vi "UI.vi"() -> ()   [LabVIEW 2016, in "中水三立SQL数据传输.lvlib"]
panel:
  out "数据大小":i32
  out "数据上传中":bool
  out "当前时间":timestamp
  out "error out":errorcluster
  out "数据查表起始时间":T1
  in  "数据补传":bool caption="确定"
  out "读取报文显示":string
  out "发送报文显示":string
  out "通信状态":bool
  in  "配置信息":T2
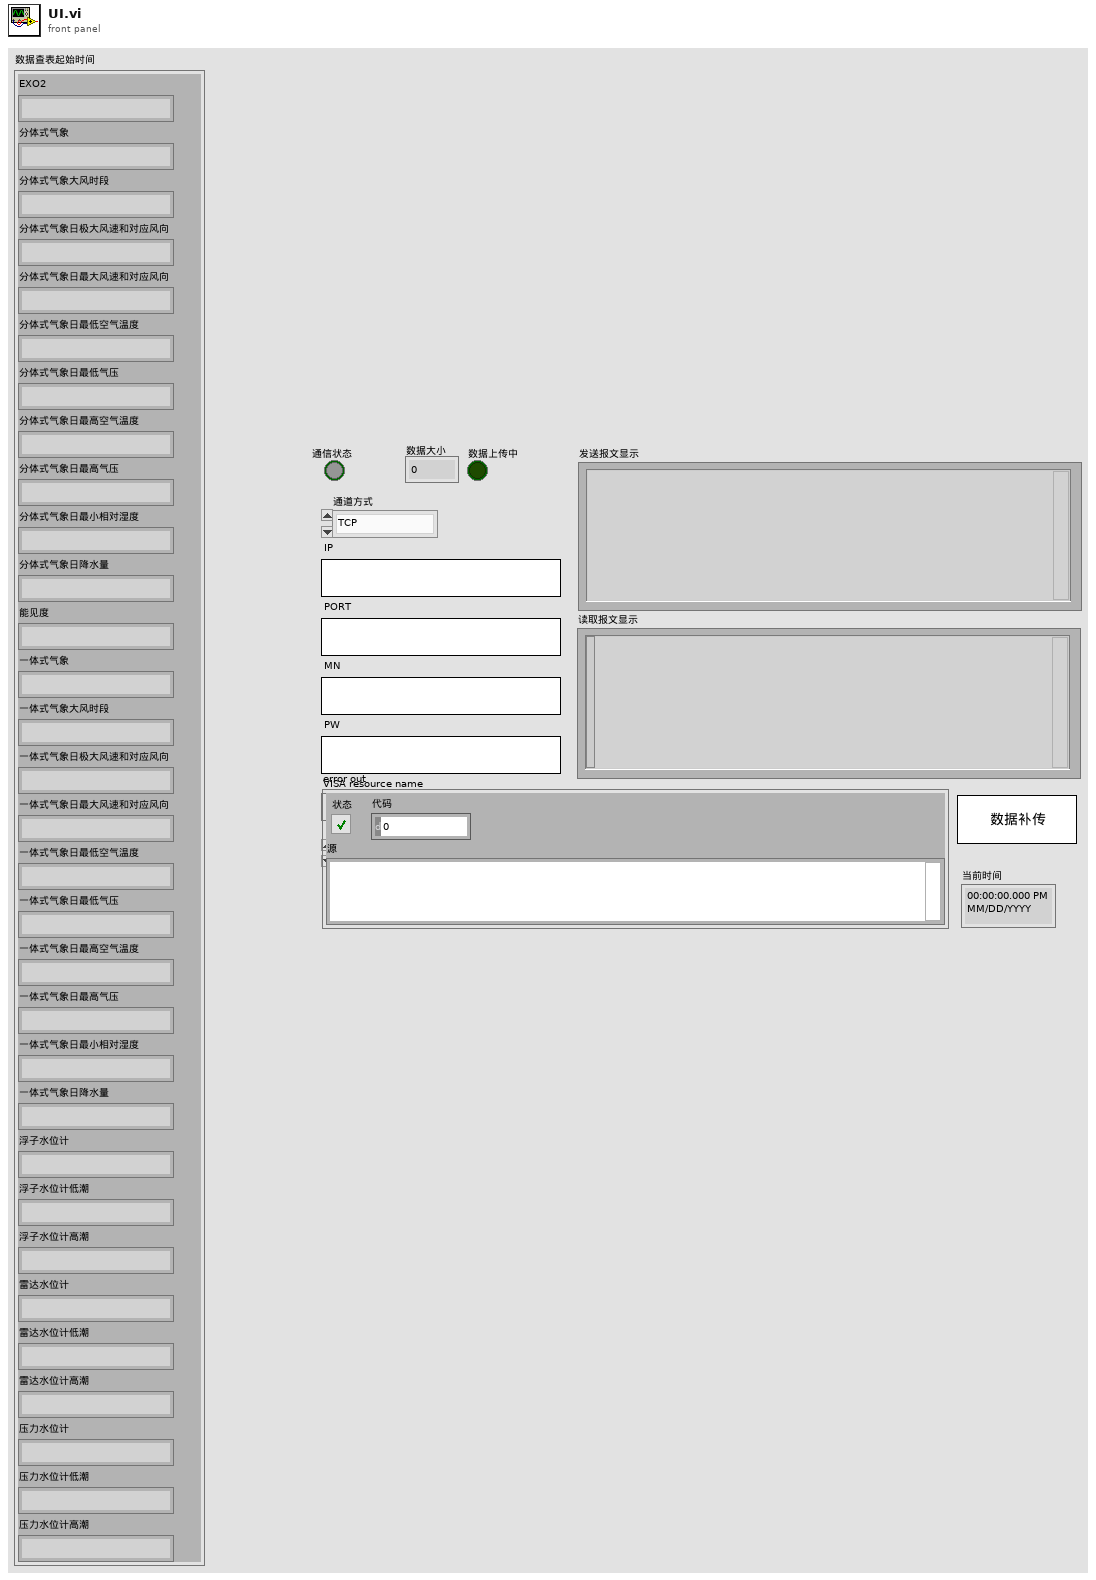
[diagram p1: front panel]
types:
  T1 = cluster{"EXO2":string, "分体式气象":string, "分体式气象大风时段":string, "分体式气象日极大风速和对应风向":string, "分体式气象日最大风速和对应风向":string, "分体式气象日最低空气温度":string, "分体式气象日最低气压":string, "分体式气象日最高空气温度":string, "分体式气象日最高气压":string, "分体式气象日最小相对湿度":string, "分体式气象日降水量":string, "能见度":string, "一体式气象":string, "一体式气象大风时段":string, "一体式气象日极大风速和对应风向":string, "一体式气象日最大风速和对应风向":string, "一体式气象日最低空气温度":string, "一体式气象日最低气压":string, "一体式气象日最高空气温度":string, "一体式气象日最高气压":string, "一体式气象日最小相对湿度":string, "一体式气象日降水量":string, "浮子水位计":string, "浮子水位计低潮":string, "浮子水位计高潮":string, "雷达水位计":string, "雷达水位计低潮":string, "雷达水位计高潮":string, "压力水位计":string, "压力水位计低潮":string, "压力水位计高潮":string}
  T2 = cluster{"通道方式":enum16{"TCP", "serial"}, "IP":string, "PORT":string, "MN":string, "PW":string, "VISA resource name":refnum<visa-resource-name>, "baud rate":u32}
  T3 = typedef "LVDateTimeRec.ctl" = cluster{"秒数的小数部分":dbl, "秒":i32, "分":i32, "时":i32, "日":i32, "月":i32, "年":i32, "天数（周）":i32, "天数（年）":i32, "DST":i32}
  T4 = cluster{"[0]":string, "[1]":string, "[2]":string, "[3]":string, "[4]":string, "[5]":string, "[6]":string, "[7]":string, "[8]":string, "[9]":string, "[10]":string, "[11]":string, "[12]":string, "[13]":string, "[14]":string, "[15]":string, "[16]":string, "[17]":string, "[18]":string, "[19]":string, "[20]":string, "[21]":string, "[22]":string, "[23]":string, "[24]":string, "[25]":string, "[26]":string, "[27]":string, "[28]":string, "[29]":string, "[30]":string}
  T5 = cluster{"枚举":enum16{"TCP", "serial"}, "IP":string, "PORT":string, "MN":string, "PW":string, "VISA resource name":refnum<visa-resource-name>, "baud rate":u32}
  T6 = cluster{"枚举":enum16{"打开连接", "发送数据", "读取数据", "数据处理", "关闭连接"}, "data":string}
  T7 = typedef "中水三立SQL数据传输.lvlib/data_in.ctl" = cluster{"PW":string, "MN":string, "table输入":T8, "数据发送次数":i32, "枚举":enum16{"返回请求应答", "上传数据", "返回执行结果"}, "type":T9, "因子编码&数据类型":cluster{"因子编码":string, "数据类型":string}[]}
  T8 = typedef "中水三立SQL数据传输.lvlib/table.ctl" = string
  T9 = typedef "中水三立SQL数据传输.lvlib/Type.ctl" = string
  T10 = cluster{"table":string, "columns":string[], "condition":string, "data_in":T7}
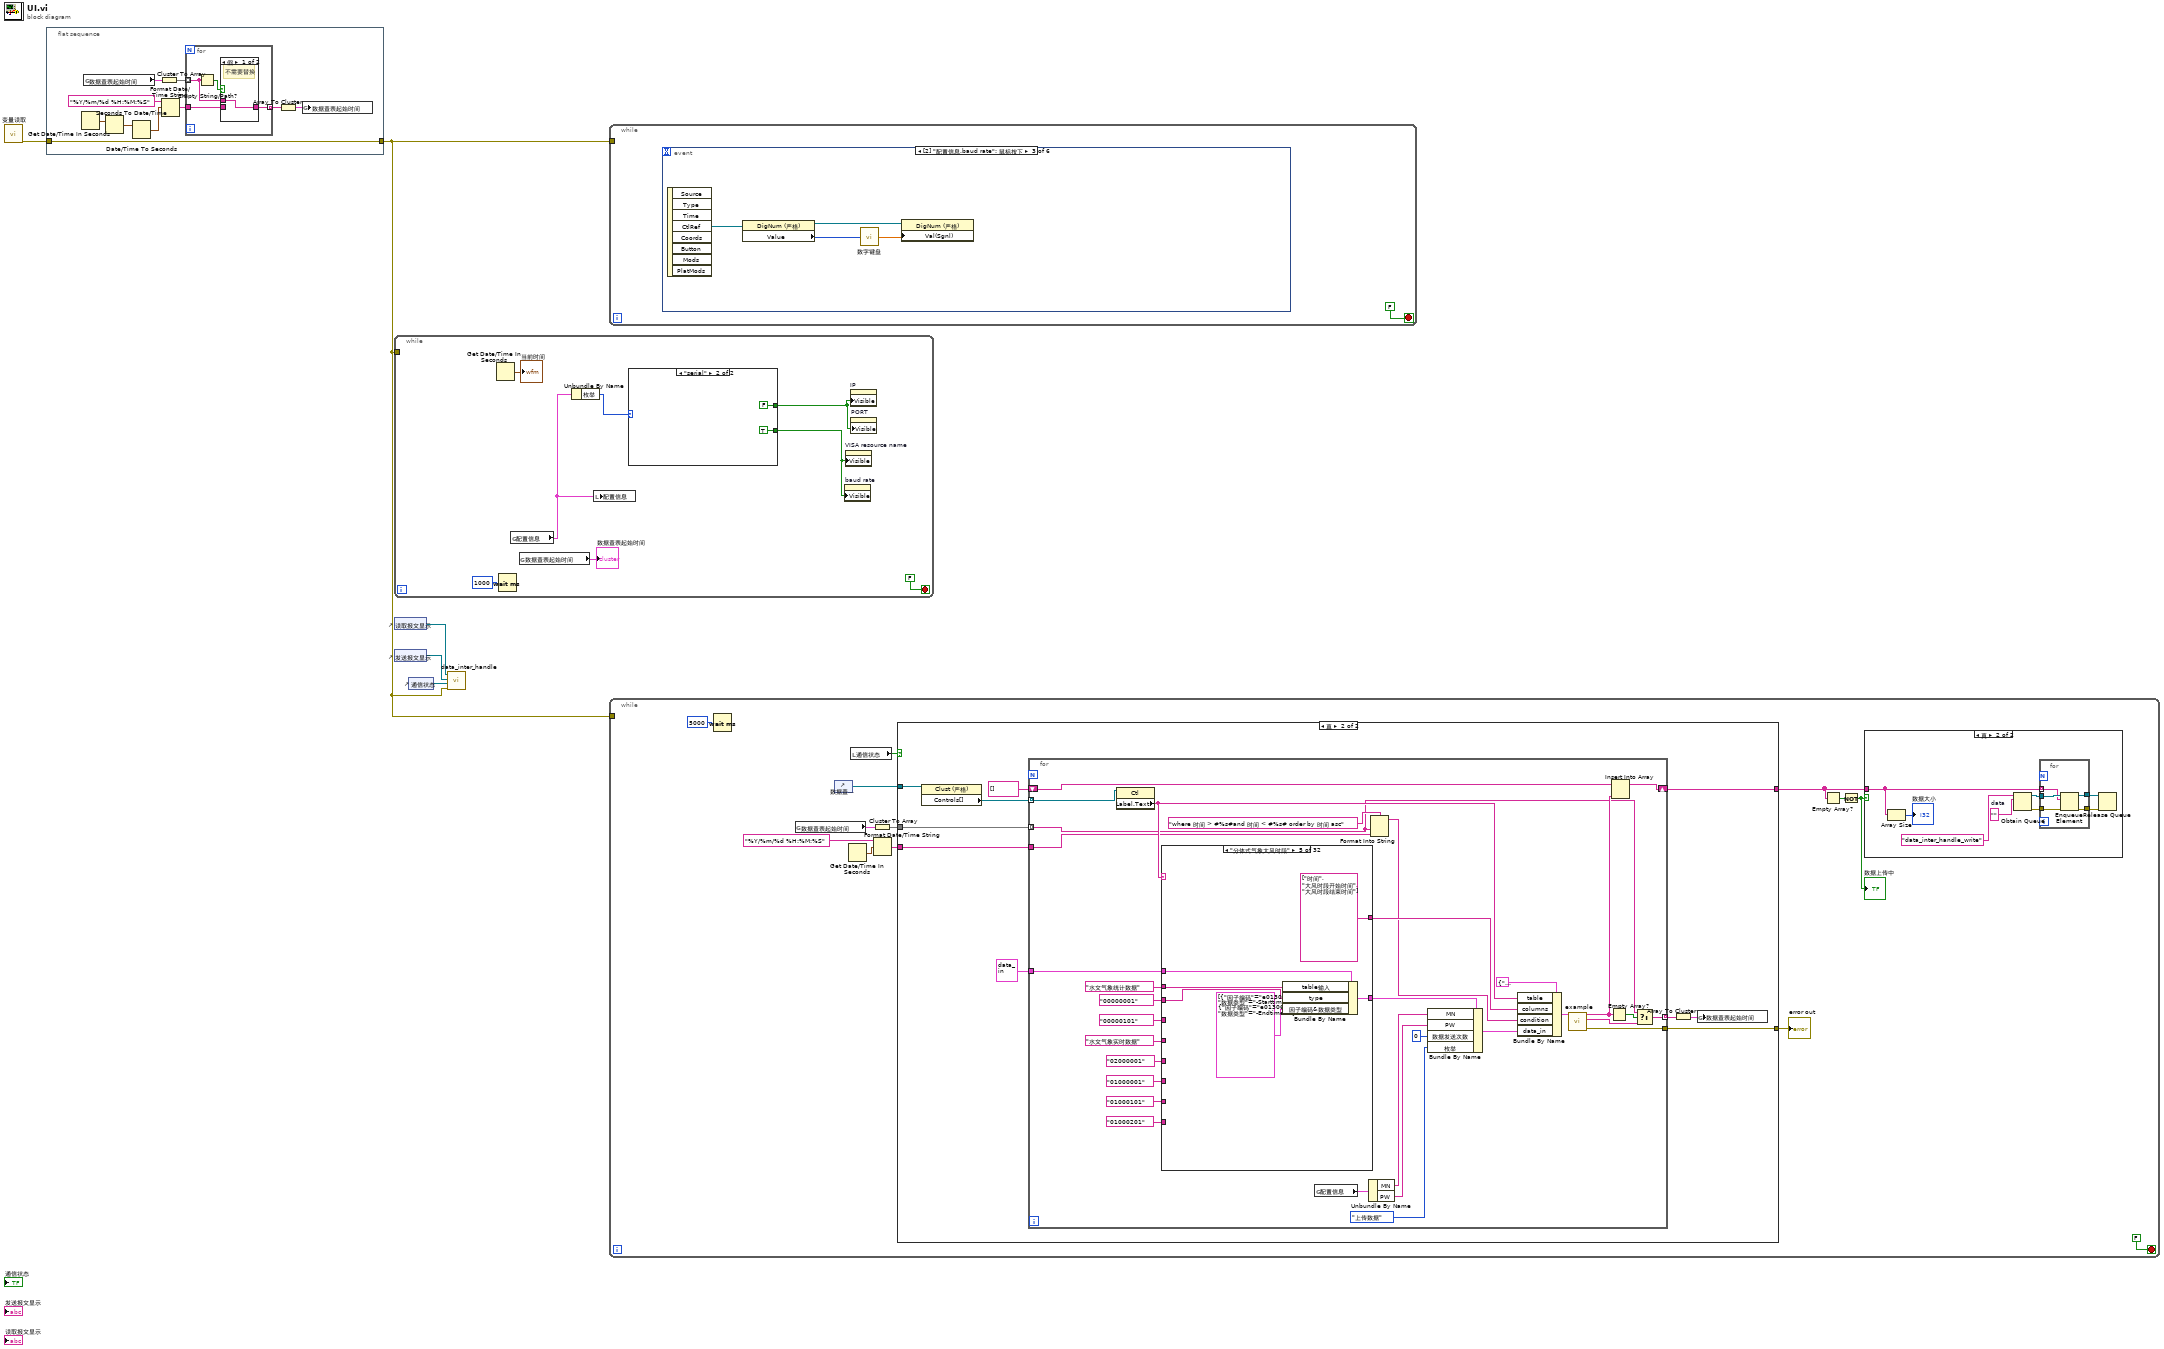
[diagram p0: block diagram]
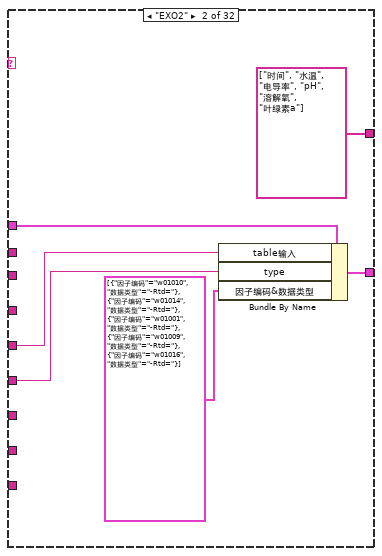
[diagram p5: hidden frame]
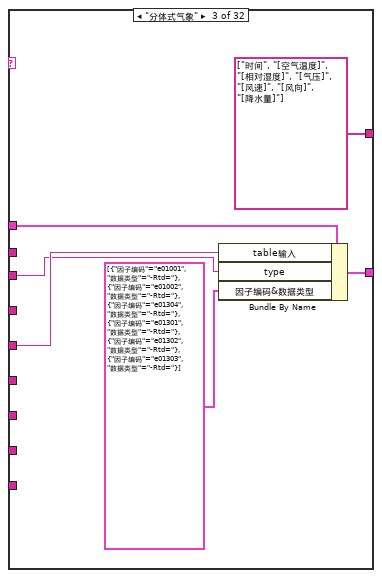
[diagram p6: hidden frame]
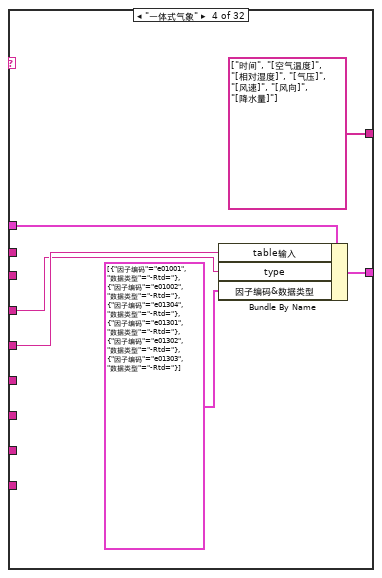
[diagram p7: hidden frame]
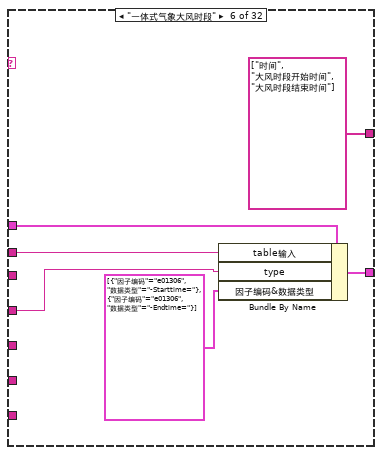
[diagram p8: hidden frame]
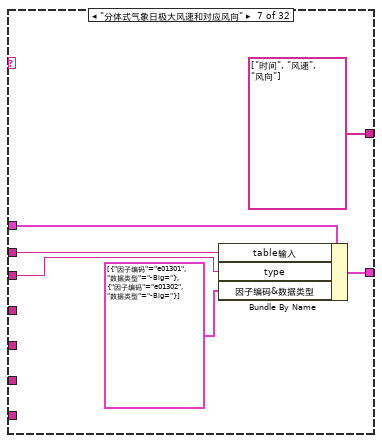
[diagram p9: hidden frame]
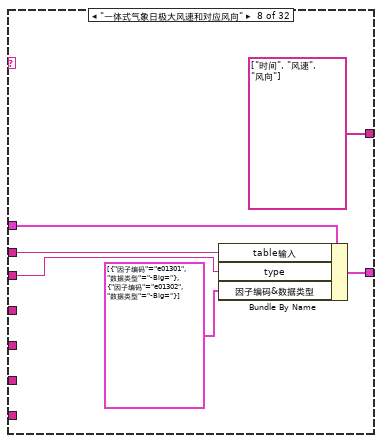
[diagram p10: hidden frame]
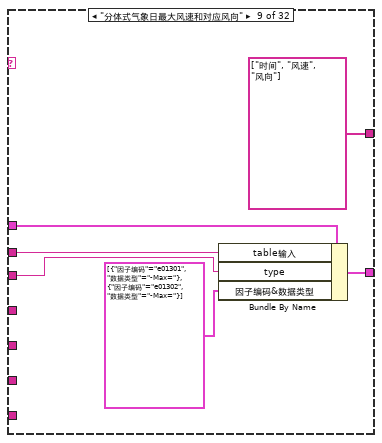
[diagram p11: hidden frame]
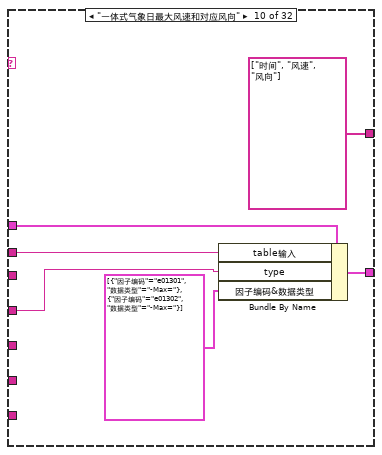
[diagram p12: hidden frame]
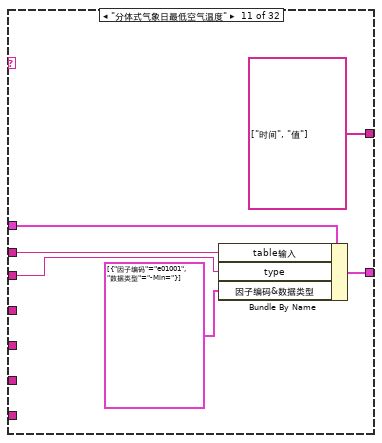
[diagram p13: hidden frame]
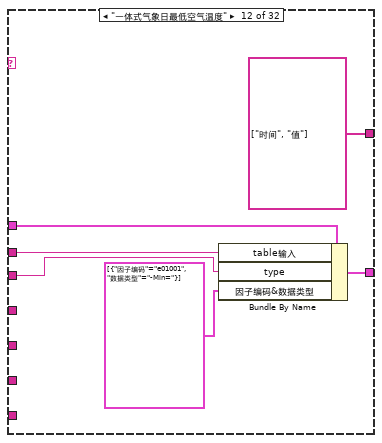
[diagram p14: hidden frame]
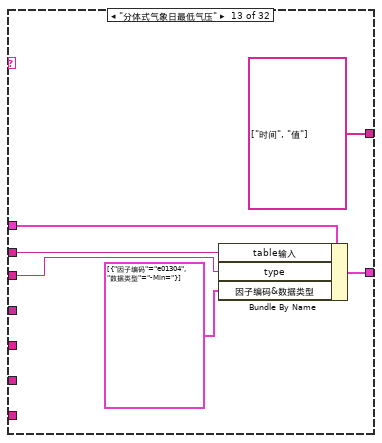
[diagram p15: hidden frame]
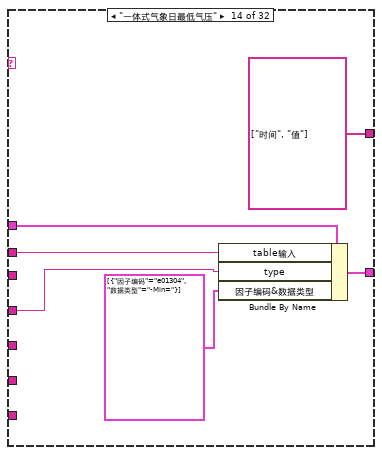
[diagram p16: hidden frame]
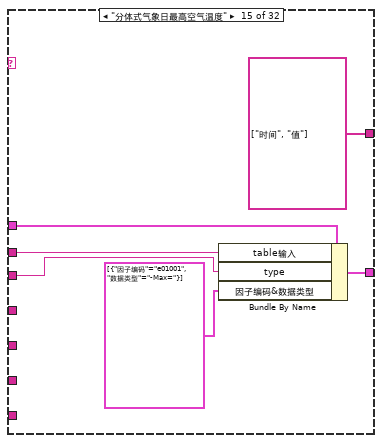
[diagram p17: hidden frame]
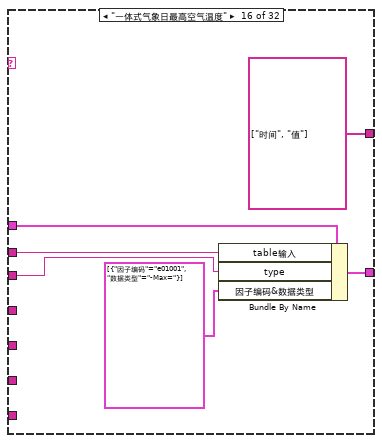
[diagram p18: hidden frame]
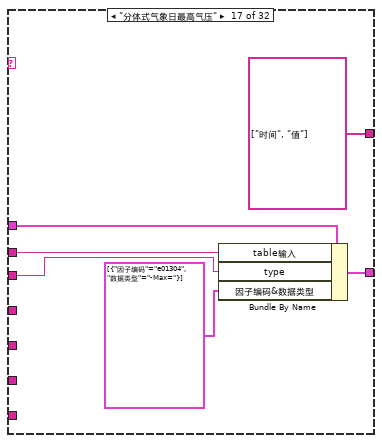
[diagram p19: hidden frame]
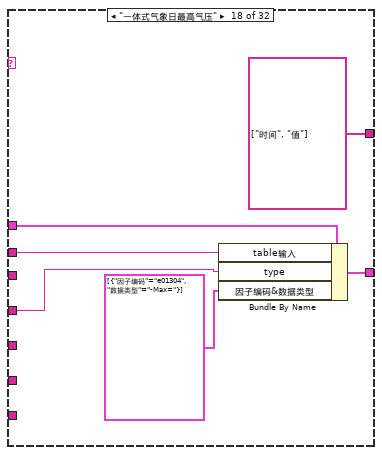
[diagram p20: hidden frame]
diagram:
  n1 = call "变量读取.vi"() -> ("错误输出"=w5:errorcluster)  [unwired: 11 in]
  n2 = flat-sequence {
    tunnel: w5 -> [w8]
    tunnel: [w8] -> w4
    frame #0 {
      n3 = Get Date/Time In Seconds() -> (seconds since 1Jan1904=w7:timestamp)
      n4 = global read "断电保存全局.vi" "数据查表起始时间"() -> (w13:cluster{"dbo.LS_Data":string})
      n5 = Seconds To Date/Time(time stamp (now)=w7) -> (date time rec=w6:T3)  [unwired: 1 in]
      n6 = Date/Time To Seconds(2:w6) -> (0:w11:timestamp)  [unwired: 1 in]
      n7 = Cluster To Array(cluster=w13) -> (array=w14:string[])
      n8 = Format Date/Time String(time format string (%c)="%Y/%m/%d %H:%M:%S" ("时间格式字符串(%c)"), seconds (now)=w11) -> (date/time string=w10:string)  [unwired: 1 in]
      n9 = for {
        tunnel: w14 -> [w16] mode=indexing
        tunnel: w10 -> [w18]
        tunnel: [w17] -> w15 mode=indexing
        n10 = Empty String/Path?(string/path=w16) -> (empty?=w19:bool)
        n11 = case shown="假" w19 {
          tunnel: w18 -> [_ w21]
          tunnel: [w20 w21] -> w17
          tunnel: w16 -> [w20 _]
          frame False {
            # "不需要替换"
          }
          frame True {
            # "空字符串，替换"
          }
        }
      }
      n12 = Array To Cluster(array=w15) -> (cluster=w9:T4)
      n13 = global write "断电保存全局.vi" "数据查表起始时间"(w9) -> ()
    }
  }
  n14 = while {
    tunnel: w4 -> [_]
    stop <- FALSE stop-if-true
    n15 = Get Date/Time In Seconds() -> (seconds since 1Jan1904=→"当前时间":timestamp)
    n16 = Wait (ms)(milliseconds to wait=u32 1000 ("等待时间（毫秒）")) -> ()  [unwired: 1 out]
    n17 = global read "断电保存全局.vi" "配置信息"() -> (w25:T5)
    n18 = global read "断电保存全局.vi" "数据查表起始时间"() -> (→"数据查表起始时间":cluster{"dbo.LS_Data":string})
    n19 = Unbundle By Name(w25) -> ("枚举"=w24:enum16{"TCP", "serial"})
    n20 = local write "配置信息"(w25) -> ()
    n21 = case shown="\"serial\"" w24 {
      tunnel: [TRUE FALSE] -> w23
      tunnel: [FALSE TRUE] -> w22
      frame "TCP", Default {
      }
      frame "serial" {
      }
    }
    n22 = property on="baud rate" class="DigNum (严格)"("Visible"=w22) -> ()  [unwired: 2 in, 2 out]
    n23 = property on="VISA resource name" class="VISAName"("Visible"=w22) -> ()  [unwired: 2 in, 2 out]
    n24 = property on="IP" class="Str"("Visible"=w23) -> ()  [unwired: 2 in, 2 out]
    n25 = property on="PORT" class="Str"("Visible"=w23) -> ()  [unwired: 2 in, 2 out]
  }
  n26 = control-ref of="读取报文显示"() -> (w2:refnum<vi>)
  n27 = control-ref of="发送报文显示"() -> (w3:refnum<vi>)
  n28 = control-ref of="通信状态"() -> (w1:refnum<vi>)
  n29 = call "data_inter_handle.vi"("error in (no error)"=w4, "通信状态"=w1, "发送报文显示"=w3, "读取报文显示"=w2) -> ()  [unwired: 7 in, 1 out]
  n30 = while {
    tunnel: w4 -> [_]
    stop <- FALSE stop-if-true
    n31 = event shown="[2] \"配置信息.baud rate\": 鼠标按下" {
      selector: _ -> [_ _ _ _ _ _]
      dyn-events: _ -> [_ _ _ _ _ _]
      timeout: _ -> [_ _ _ _ _ _]
      event Timeout {
        n32 = event-data() -> ()  [unwired: 1 in, 3 out]
      }
      event "配置信息.IP", "配置信息.PORT": Mouse Down {
        n33 = event-data() -> ("CtlRef"=w43:refnum<vi>)  [unwired: 1 in, 7 out]
        n34 = property class="Str"(reference=w43) -> (reference out=w36:refnum<vi>, "Value"=w42:string)  [unwired: 1 in, 1 out]
        n35 = call "IP键盘.vi"("OldNumber"=w42) -> ("NewNumber"=w35:string)
        n36 = String Length(string=w35) -> (length=w41:i32)
        n37 = Less Or Equal?(x=w41, y=50) -> (x <= y?=w39:bool)
        n38 = case shown="假" w39 {
          tunnel: w36 -> [w44 w48]
          tunnel: w35 -> [_ w47]
          tunnel: [w44 w48] -> w38
          tunnel: ["127.0.0.1" w47] -> w37
          frame False {
            n39 = One Button Dialog(message="超过ipv4最大长度限制,请重新输入!" ("消息")) -> ()  [unwired: 1 in, 1 out]
          }
          frame True {
          }
        }
        n40 = property class="Str"(reference=w38, "Val(Sgnl)"=w37) -> ()  [unwired: 1 in, 2 out]
      }
      event "配置信息.baud rate": Mouse Down {
        n41 = event-data() -> ("CtlRef"=w52:refnum<vi>)  [unwired: 1 in, 7 out]
        n42 = property class="DigNum (严格)"(reference=w52) -> (reference out=w50:refnum<vi>, "Value"=w51:u32)  [unwired: 1 in, 1 out]
        n43 = call "数字键盘.vi"("OldNumber"=w51) -> ("NewNumber"=w49:sgl)
        n44 = property class="DigNum (严格)"(reference=w50, "Val(Sgnl)"=w49) -> ()  [unwired: 1 in, 2 out]
      }
      event "配置信息": Value Change {
        n45 = event-data() -> ()  [unwired: 1 in, 6 out]
        n46 = flat-sequence {
          frame #0 {
            n47 = global write "断电保存全局.vi" "配置信息"("配置信息") -> ()
          }
          frame #1 {
            w58 = T6 {"枚举"=enum."打开连接", "data"=""}
            n48 = call "变量存储.vi"() -> ()  [unwired: 12 in]
            n49 = Bundle By Name(cluster=w58, "枚举"=enum16{"打开连接", "发送数据", "读取数据", "数据处理", "关闭连接"}."关闭连接") -> (w57:T6)
            n50 = Obtain Queue(name (unnamed)="data_inter_handle" ("名称（未命名）"), element data type=w58) -> (queue out=w60:refnum<queue>, error out=w59:errorcluster)  [unwired: 3 in, 1 out]
            n51 = Enqueue Element(queue=w60, element=w57, error in (no error)=w59) -> (queue out=w54:refnum<queue>, error out=w55:errorcluster)  [unwired: 1 in, 1 out]
            n52 = Release Queue(queue=w54, error in (no error)=w55) -> ()  [unwired: 1 in, 3 out]
          }
        }
      }
      event "数据补传": Value Change {
        n53 = event-data() -> ()  [unwired: 1 in, 6 out]
        n54 = call "数据补传对话框.vi"() -> ("输出"=w63:bool, "时间OUT"=w62:timestamp)  [unwired: 10 in]
        n55 = case shown="真" w63 {
          tunnel: w62 -> [_ w68]
          frame False {
          }
          frame True {
            n56 = Format Date/Time String(time format string (%c)="%Y/%m/%d %H:%M:%S" ("时间格式字符串(%c)"), seconds (now)=w68) -> (date/time string=w65:string)  [unwired: 1 in]
            n57 = Initialize Array(w65, 31 ("维数大小")) -> (w64:string[])
            n58 = Array To Cluster(array=w64) -> (cluster=w66:T4)
            n59 = global write "断电保存全局.vi" "数据查表起始时间"(w66) -> ()
          }
        }
      }
      event Panel Close {
        n60 = event-data() -> ()  [unwired: 1 in, 4 out]
        n61 = Quit LabVIEW(quit? (T)=TRUE ("退出？(T)")) -> ()
      }
    }
  }
  n62 = while {
    tunnel: w4 -> [_]
    stop <- FALSE stop-if-true
    n63 = Wait (ms)(milliseconds to wait=u32 5000 ("等待时间（毫秒）")) -> ()  [unwired: 1 out]
    n64 = global read "断电保存全局.vi" "数据查表起始时间"() -> (w81:cluster{"dbo.LS_Data":string})
    n65 = control-ref of="数据查表起始时间"() -> (w75:refnum<vi>)
    n66 = Get Date/Time In Seconds() -> (seconds since 1Jan1904=w77:timestamp)
    n67 = local read "通信状态"() -> (w72:bool)
    n68 = Cluster To Array(cluster=w81) -> (array=w80:string[])
    n69 = Format Date/Time String(time format string (%c)="%Y/%m/%d %H:%M:%S" ("时间格式字符串(%c)"), seconds (now)=w77) -> (date/time string=w78:string)  [unwired: 1 in]
    n70 = case shown="真" w72 {
      tunnel: w80 -> [_ w93]
      tunnel: w78 -> [_ w92]
      tunnel: [_ w91] -> w71
      tunnel: w75 -> [_ w90]
      tunnel: [_ w88] -> w74
      frame False {
      }
      frame True {
        n71 = property class="Clust (严格)"(reference=w90) -> ("Controls[]"=w89:refnum<vi>[])  [unwired: 1 in, 2 out]
        n72 = for {
          tunnel: w93 -> [w108] mode=indexing
          tunnel: w89 -> [w125] mode=indexing
          tunnel: w92 -> [w114]
          shift-right: [w111] -> w91
          shift-left: string[] [] ("message") -> [w112]
          tunnel: [w106] -> w85 mode=indexing
          tunnel: [w105] -> w88
          tunnel: T7 {"PW"="123456", "MN"="TEST001", "table输入"="心跳包", "数据发送次数"=0, "枚举"=enum."上传数据", "type"="00000001", "因子编码&数据类型"=[{"因子编码"="e01306", "数据类型"="-Starttime="}, {"因子编码"="e01307", "数据类型"="-Endtime="}]} ("data_in") -> [w103]
          n73 = property class="Ctl"(reference=w125) -> ("Label.Text"=w124:string)  [unwired: 1 in, 2 out]
          n74 = case shown="\"分体式气象大风时段\"" w124 {
            tunnel: [_ string[] ["时间", "水温", "电导率", "pH", "溶解氧", "叶绿素a"] ("columns") string[] ["时间", "[空气温度]", "[相对湿度]", "[气压]", "[风速]", "[风向]", "[降水量]"] ("columns") string[] ["时间", "[空气温度]", "[相对湿度]", "[气压]", "[风速]", "[风向]", "[降水量]"] ("columns") string[] ["时间", "大风时段开始时间", "大风时段结束时间"] ("columns") string[] ["时间", "大风时段开始时间", "大风时段结束时间"] ("columns") string[] ["时间", "风速", "风向"] ("columns") string[] ["时间", "风速", "风向"] ("columns") string[] ["时间", "风速", "风向"] ("columns") string[] ["时间", "风速", "风向"] ("columns") string[] ["时间", "值"] ("columns") string[] ["时间", "值"] ("columns") string[] ["时间", "值"] ("columns") string[] ["时间", "值"] ("columns") string[] ["时间", "值"] ("columns") string[] ["时间", "值"] ("columns") string[] ["时间", "值"] ("columns") string[] ["时间", "值"] ("columns") string[] ["时间", "值"] ("columns") string[] ["时间", "值"] ("columns") string[] ["时间", "值"] ("columns") string[] ["时间", "值"] ("columns") string[] ["时间", "[60秒能见度]"] ("columns") string[] ["时间", "[潮高]"] ("columns") string[] ["时间", "[潮高]"] ("columns") string[] ["时间", "[潮高]"] ("columns") string[] ["时间", "[潮高]"] ("columns") string[] ["时间", "[潮高]"] ("columns") string[] ["时间", "[潮高]"] ("columns") string[] ["时间", "[潮高]"] ("columns") string[] ["时间", "[潮高]"] ("columns") string[] ["时间", "[潮高]"] ("columns")] -> w123
            tunnel: w103 -> [_ w130 w136 w142 w148 w154 w160 w166 w172 w178 w184 w190 w196 w202 w208 w214 w220 w226 w232 w238 w244 w250 w256 w262 w268 w274 w280 w286 w292 w298 w304 w310]
            tunnel: [_ w129 w135 w141 w147 w153 w159 w165 w171 w177 w183 w189 w195 w201 w207 w213 w219 w225 w231 w237 w243 w249 w255 w261 w267 w273 w279 w285 w291 w297 w303 w309] -> w122
            tunnel: T9 "00000001" ("type") -> [_ _ w132 _ w145 _ w157 w162 w169 _ w181 w187 w193 _ w205 w211 w217 _ w229 _ w240 _ w252 _ _ _ _ _ _ _ _ _]
            tunnel: T9 "00000101" ("type") -> [_ _ _ w138 _ w150 _ _ _ w175 _ _ _ w199 _ _ _ w223 _ w235 _ w247 _ _ _ _ _ _ _ _ _ _]
            tunnel: T9 "01000001" ("type") -> [_ _ _ _ _ _ _ _ _ _ _ _ _ _ _ _ _ _ _ _ _ _ _ w259 _ _ w276 _ _ w295 _ _]
            tunnel: T9 "01000101" ("type") -> [_ _ _ _ _ _ _ _ _ _ _ _ _ _ _ _ _ _ _ _ _ _ _ _ w265 _ _ w283 _ _ w300 _]
            tunnel: T9 "01000201" ("type") -> [_ _ _ _ _ _ _ _ _ _ _ _ _ _ _ _ _ _ _ _ _ _ _ _ _ w271 _ _ w288 _ _ w307]
            tunnel: T9 "02000001" ("type") -> [_ w126 _ _ _ _ _ _ _ _ _ _ _ _ _ _ _ _ _ _ _ _ _ _ _ _ _ _ _ _ _ _]
            tunnel: T8 "水文气象实时数据" ("table输入") -> [_ w127 w133 w139 _ _ _ _ _ _ _ _ _ _ _ _ _ _ _ _ _ _ w253 w258 w264 w270 _ _ _ _ _ _]
            tunnel: T8 "水文气象统计数据" ("table输入") -> [_ _ _ _ w144 w151 w156 w163 w168 w174 w180 w186 w192 w198 w204 w210 w216 w222 w228 w234 w241 w246 _ _ _ _ w277 w282 w289 w294 w301 w306]
            frame "假", Default {
            }
            frame "EXO2" {
              n75 = Bundle By Name(cluster=w130, "table输入"=w127, "type"=w126, "因子编码&数据类型"=cluster{"因子编码":string, "数据类型":string}[] [{"因子编码"="w01010", "数据类型"="-Rtd="}, {"因子编码"="w01014", "数据类型"="-Rtd="}, {"因子编码"="w01001", "数据类型"="-Rtd="}, {"因子编码"="w01009", "数据类型"="-Rtd="}, {"因子编码"="w01016", "数据类型"="-Rtd="}]) -> (w129:T7)
            }
            frame "分体式气象" {
              n76 = Bundle By Name(cluster=w136, "table输入"=w133, "type"=w132, "因子编码&数据类型"=cluster{"因子编码":string, "数据类型":string}[] [{"因子编码"="e01001", "数据类型"="-Rtd="}, {"因子编码"="e01002", "数据类型"="-Rtd="}, {"因子编码"="e01304", "数据类型"="-Rtd="}, {"因子编码"="e01301", "数据类型"="-Rtd="}, {"因子编码"="e01302", "数据类型"="-Rtd="}, {"因子编码"="e01303", "数据类型"="-Rtd="}]) -> (w135:T7)
            }
            frame "一体式气象" {
              n77 = Bundle By Name(cluster=w142, "table输入"=w139, "type"=w138, "因子编码&数据类型"=cluster{"因子编码":string, "数据类型":string}[] [{"因子编码"="e01001", "数据类型"="-Rtd="}, {"因子编码"="e01002", "数据类型"="-Rtd="}, {"因子编码"="e01304", "数据类型"="-Rtd="}, {"因子编码"="e01301", "数据类型"="-Rtd="}, {"因子编码"="e01302", "数据类型"="-Rtd="}, {"因子编码"="e01303", "数据类型"="-Rtd="}]) -> (w141:T7)
            }
            frame "分体式气象大风时段" {
              n78 = Bundle By Name(cluster=w148, "table输入"=w144, "type"=w145, "因子编码&数据类型"=cluster{"因子编码":string, "数据类型":string}[] [{"因子编码"="e01306", "数据类型"="-Starttime="}, {"因子编码"="e01306", "数据类型"="-Endtime="}]) -> (w147:T7)
            }
            frame "一体式气象大风时段" {
              n79 = Bundle By Name(cluster=w154, "table输入"=w151, "type"=w150, "因子编码&数据类型"=cluster{"因子编码":string, "数据类型":string}[] [{"因子编码"="e01306", "数据类型"="-Starttime="}, {"因子编码"="e01306", "数据类型"="-Endtime="}]) -> (w153:T7)
            }
            frame "分体式气象日极大风速和对应风向" {
              n80 = Bundle By Name(cluster=w160, "table输入"=w156, "type"=w157, "因子编码&数据类型"=cluster{"因子编码":string, "数据类型":string}[] [{"因子编码"="e01301", "数据类型"="-Big="}, {"因子编码"="e01302", "数据类型"="-Big="}]) -> (w159:T7)
            }
            frame "一体式气象日极大风速和对应风向" {
              n81 = Bundle By Name(cluster=w166, "table输入"=w163, "type"=w162, "因子编码&数据类型"=cluster{"因子编码":string, "数据类型":string}[] [{"因子编码"="e01301", "数据类型"="-Big="}, {"因子编码"="e01302", "数据类型"="-Big="}]) -> (w165:T7)
            }
            frame "分体式气象日最大风速和对应风向" {
              n82 = Bundle By Name(cluster=w172, "table输入"=w168, "type"=w169, "因子编码&数据类型"=cluster{"因子编码":string, "数据类型":string}[] [{"因子编码"="e01301", "数据类型"="-Max="}, {"因子编码"="e01302", "数据类型"="-Max="}]) -> (w171:T7)
            }
            frame "一体式气象日最大风速和对应风向" {
              n83 = Bundle By Name(cluster=w178, "table输入"=w174, "type"=w175, "因子编码&数据类型"=cluster{"因子编码":string, "数据类型":string}[] [{"因子编码"="e01301", "数据类型"="-Max="}, {"因子编码"="e01302", "数据类型"="-Max="}]) -> (w177:T7)
            }
            frame "分体式气象日最低空气温度" {
              n84 = Bundle By Name(cluster=w184, "table输入"=w180, "type"=w181, "因子编码&数据类型"=cluster{"因子编码":string, "数据类型":string}[] [{"因子编码"="e01001", "数据类型"="-Min="}]) -> (w183:T7)
            }
            frame "一体式气象日最低空气温度" {
              n85 = Bundle By Name(cluster=w190, "table输入"=w186, "type"=w187, "因子编码&数据类型"=cluster{"因子编码":string, "数据类型":string}[] [{"因子编码"="e01001", "数据类型"="-Min="}]) -> (w189:T7)
            }
            frame "分体式气象日最低气压" {
              n86 = Bundle By Name(cluster=w196, "table输入"=w192, "type"=w193, "因子编码&数据类型"=cluster{"因子编码":string, "数据类型":string}[] [{"因子编码"="e01304", "数据类型"="-Min="}]) -> (w195:T7)
            }
            frame "一体式气象日最低气压" {
              n87 = Bundle By Name(cluster=w202, "table输入"=w198, "type"=w199, "因子编码&数据类型"=cluster{"因子编码":string, "数据类型":string}[] [{"因子编码"="e01304", "数据类型"="-Min="}]) -> (w201:T7)
            }
            frame "分体式气象日最高空气温度" {
              n88 = Bundle By Name(cluster=w208, "table输入"=w204, "type"=w205, "因子编码&数据类型"=cluster{"因子编码":string, "数据类型":string}[] [{"因子编码"="e01001", "数据类型"="-Max="}]) -> (w207:T7)
            }
            frame "一体式气象日最高空气温度" {
              n89 = Bundle By Name(cluster=w214, "table输入"=w210, "type"=w211, "因子编码&数据类型"=cluster{"因子编码":string, "数据类型":string}[] [{"因子编码"="e01001", "数据类型"="-Max="}]) -> (w213:T7)
            }
            frame "分体式气象日最高气压" {
              n90 = Bundle By Name(cluster=w220, "table输入"=w216, "type"=w217, "因子编码&数据类型"=cluster{"因子编码":string, "数据类型":string}[] [{"因子编码"="e01304", "数据类型"="-Max="}]) -> (w219:T7)
            }
            frame "一体式气象日最高气压" {
              n91 = Bundle By Name(cluster=w226, "table输入"=w222, "type"=w223, "因子编码&数据类型"=cluster{"因子编码":string, "数据类型":string}[] [{"因子编码"="e01304", "数据类型"="-Max="}]) -> (w225:T7)
            }
            frame "分体式气象日最小相对湿度" {
              n92 = Bundle By Name(cluster=w232, "table输入"=w228, "type"=w229, "因子编码&数据类型"=cluster{"因子编码":string, "数据类型":string}[] [{"因子编码"="e01002", "数据类型"="-Min="}]) -> (w231:T7)
            }
            frame "一体式气象日最小相对湿度" {
              n93 = Bundle By Name(cluster=w238, "table输入"=w234, "type"=w235, "因子编码&数据类型"=cluster{"因子编码":string, "数据类型":string}[] [{"因子编码"="e01002", "数据类型"="-Min="}]) -> (w237:T7)
            }
            frame "分体式气象日降水量" {
              n94 = Bundle By Name(cluster=w244, "table输入"=w241, "type"=w240, "因子编码&数据类型"=cluster{"因子编码":string, "数据类型":string}[] [{"因子编码"="e01303", "数据类型"="-Day="}]) -> (w243:T7)
            }
            frame "一体式气象日降水量" {
              n95 = Bundle By Name(cluster=w250, "table输入"=w246, "type"=w247, "因子编码&数据类型"=cluster{"因子编码":string, "数据类型":string}[] [{"因子编码"="e01303", "数据类型"="-Day="}]) -> (w249:T7)
            }
            frame "能见度" {
              n96 = Bundle By Name(cluster=w256, "table输入"=w253, "type"=w252, "因子编码&数据类型"=cluster{"因子编码":string, "数据类型":string}[] [{"因子编码"="e01305", "数据类型"="-Rtd="}]) -> (w255:T7)
            }
            frame "浮子水位计" {
              n97 = Bundle By Name(cluster=w262, "table输入"=w258, "type"=w259, "因子编码&数据类型"=cluster{"因子编码":string, "数据类型":string}[] [{"因子编码"="e01308", "数据类型"="-Rtd="}]) -> (w261:T7)
            }
            frame "雷达水位计" {
              n98 = Bundle By Name(cluster=w268, "table输入"=w264, "type"=w265, "因子编码&数据类型"=cluster{"因子编码":string, "数据类型":string}[] [{"因子编码"="e01308", "数据类型"="-Rtd="}]) -> (w267:T7)
            }
            frame "压力水位计" {
              n99 = Bundle By Name(cluster=w274, "table输入"=w270, "type"=w271, "因子编码&数据类型"=cluster{"因子编码":string, "数据类型":string}[] [{"因子编码"="e01308", "数据类型"="-Rtd="}]) -> (w273:T7)
            }
            frame "浮子水位计低潮" {
              n100 = Bundle By Name(cluster=w280, "table输入"=w277, "type"=w276, "因子编码&数据类型"=cluster{"因子编码":string, "数据类型":string}[] [{"因子编码"="e01310", "数据类型"="-Trough="}]) -> (w279:T7)
            }
            frame "雷达水位计低潮" {
              n101 = Bundle By Name(cluster=w286, "table输入"=w282, "type"=w283, "因子编码&数据类型"=cluster{"因子编码":string, "数据类型":string}[] [{"因子编码"="e01310", "数据类型"="-Trough="}]) -> (w285:T7)
            }
            frame "压力水位计低潮" {
              n102 = Bundle By Name(cluster=w292, "table输入"=w289, "type"=w288, "因子编码&数据类型"=cluster{"因子编码":string, "数据类型":string}[] [{"因子编码"="e01310", "数据类型"="-Trough="}]) -> (w291:T7)
            }
            frame "浮子水位计高潮" {
              n103 = Bundle By Name(cluster=w298, "table输入"=w294, "type"=w295, "因子编码&数据类型"=cluster{"因子编码":string, "数据类型":string}[] [{"因子编码"="e01309", "数据类型"="-Peak="}]) -> (w297:T7)
            }
            frame "雷达水位计高潮" {
              n104 = Bundle By Name(cluster=w304, "table输入"=w301, "type"=w300, "因子编码&数据类型"=cluster{"因子编码":string, "数据类型":string}[] [{"因子编码"="e01309", "数据类型"="-Peak="}]) -> (w303:T7)
            }
            frame "压力水位计高潮" {
              n105 = Bundle By Name(cluster=w310, "table输入"=w306, "type"=w307, "因子编码&数据类型"=cluster{"因子编码":string, "数据类型":string}[] [{"因子编码"="e01309", "数据类型"="-Peak="}]) -> (w309:T7)
            }
          }
          n106 = global read "断电保存全局.vi" "配置信息"() -> (w121:T5)
          n107 = Unbundle By Name(w121) -> ("MN"=w120:string, "PW"=w119:string)
          n108 = Format Into String(format string="where 时间 > #%s#and 时间 < #%s# order by 时间 asc" ("初始字符串"), w108, w114) -> (resulting string=w113:string)  [unwired: 2 in, 1 out]
          n109 = Bundle By Name(cluster=w122, "MN"=w120, "PW"=w119, "数据发送次数"=0, "枚举"=enum16{"返回请求应答", "上传数据", "返回执行结果"}."上传数据") -> (w116:T7)
          n110 = Bundle By Name(cluster=T10 {"table"="分体式气象大风时段", "columns"=["时间", "大风时段开始时间", "大风时段结束时间"], "condition"="", "data_in"={"PW"="123456", "MN"="TEST001", "table输入"="心跳包", "数据发送次数"=0, "枚举"=enum."上传数据", "type"="00000001", "因子编码&数据类型"=[{"因子编码"="e01306", "数据类型"="-Starttime="}, {"因子编码"="e01307", "数据类型"="-Endtime="}]}} ("data_in"), "table"=w124, "columns"=w123, "condition"=w113, "data_in"=w116) -> (w94:T10)
          n111 = call "example.vi"("data_in"=w94) -> ("error out"=w105:errorcluster, "最新时间"=w107:string, "message"=w110:string[])  [unwired: 8 in]
          n112 = Empty Array?(array=w110) -> (empty?=w109:bool)
          n113 = Insert Into Array(array=w112, new element=w110) -> (w111:string[])  [unwired: 1 in]
          n114 = Select(t=w108, s=w109, f=w107) -> (s? t:f=w106:string)
        }
        n115 = Array To Cluster(array=w85) -> (cluster=w86:T4)
        n116 = global write "断电保存全局.vi" "数据查表起始时间"(w86) -> ()
      }
    }
    "error out" <- w74
    n117 = Empty Array?(array=w71) -> (empty?=w76:bool)
    n118 = Not(x=w76) -> (.not. x?=w73:bool)
    "数据上传中" <- w73
    n119 = case shown="真" w73 {
      tunnel: w71 -> [_ w312]
      frame False {
      }
      frame True {
        w314 = ""  # data
        n120 = Array Size(array=w312) -> (size(s)=→"数据大小":i32)
        n121 = Obtain Queue(name (unnamed)="data_inter_handle_write" ("名称（未命名）"), element data type=w314) -> (queue out=w319:refnum<queue>, error out=w318:errorcluster)  [unwired: 3 in, 1 out]
        n122 = for {
          tunnel: w319 -> [w324]
          tunnel: w318 -> [w323]
          tunnel: [w322] -> w317
          tunnel: [w321] -> w316
          tunnel: w312 -> [w320] mode=indexing
          n123 = Enqueue Element(queue=w324, element=w320, error in (no error)=w323) -> (queue out=w322:refnum<queue>, error out=w321:errorcluster)  [unwired: 1 in, 1 out]
        }
        n124 = Release Queue(queue=w317, error in (no error)=w316) -> ()  [unwired: 1 in, 3 out]
      }
    }
  }
